vi "03-without_args_and_returned_val.vi"() -> ()   [LabVIEW 2018, in "LV2Julia_examples.lvlib"]
uses:
  LV2Julia_examples.lvlib
  LV2Julia_core/VIs/Server or client state.ctl
  LV2Julia_core/VIs/detailed error info.ctl
  LV2Julia_core/VIs/StackFrame.ctl
  LV2Julia_core/VIs/Commands.ctl
  3a82b6dd-e193-42c5-8b03-f24c274193dd.vi
  3a82b6dd-e193-42c5-8b03-f24c274193dd.vi/3e2a5918-f46e-4ed7-8eb4-9a38b8d3556b.vi
  3a82b6dd-e193-42c5-8b03-f24c274193dd.vi/3e2a5918-f46e-4ed7-8eb4-9a38b8d3556b.vi/37087407-fbe7-4cab-bfef-745450405fa8.vi
  3a82b6dd-e193-42c5-8b03-f24c274193dd.vi/3e2a5918-f46e-4ed7-8eb4-9a38b8d3556b.vi/0226fe71-458f-479f-9501-f13c7d1721aa.vi
  3a82b6dd-e193-42c5-8b03-f24c274193dd.vi/3e2a5918-f46e-4ed7-8eb4-9a38b8d3556b.vi/25bfc6ec-1543-4893-b8db-c428feecb175.vi
  LV2Julia_core/VIs/jl-scripts path.vi
  LV2Julia_core/VIs/check ID validity.vi
  LV2Julia_core/VIs/bindata_descr to JSON.vi
  LV2Julia_core/VIs/check cluster field names.vi
  LV2Julia_core/VIs/concat JSON.vi
  LV2Julia_core/VIs/build request.vi
  LV2Julia_core/VIs/Parse server response.vi
  LV2Julia_core/VIs/log jl exceptions.vi
  LV2Julia_core/LV2Julia_core.lvlib
panel:
  in  "next":bool
  out "detailed error info":T1
  out "current error":errorcluster
  out "final error":errorcluster
  out "short err code":u8
  in  "stop":bool
  out "ZMQ timeout":bool
  out "Julia script file path":path
  out "temporary script path":path
  out "Jl Server state":T3
  # "No arguments are sent and no values recieved here. The Julia script should each time print \"Hello World!\" in the terminal window."
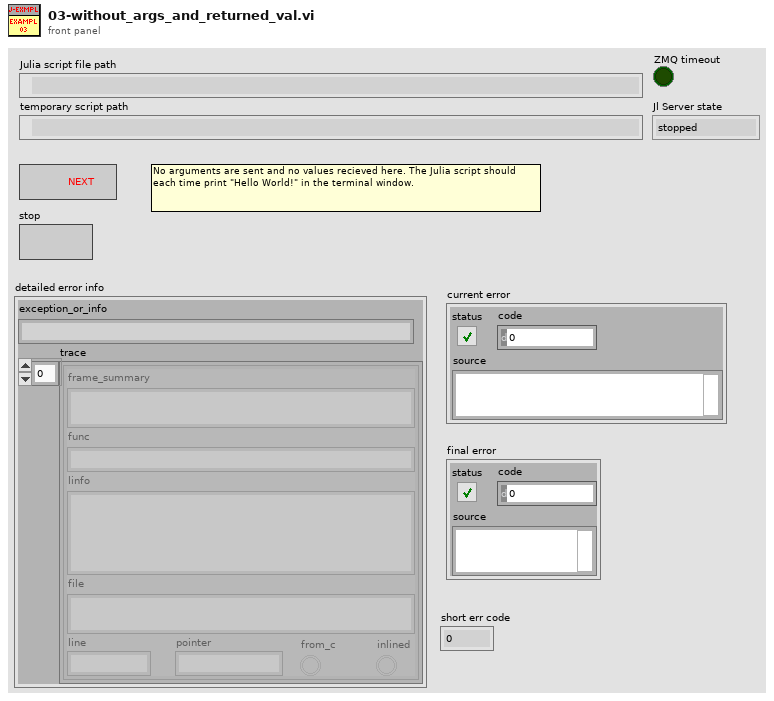
[diagram p1: front panel]
types:
  T1 = typedef "LV2Julia_core.lvlib/detailed error info.ctl" = cluster{"exception_or_info":string, "trace":T2[]}
  T2 = typedef "LV2Julia_core.lvlib/StackFrame.ctl" = cluster{"frame_summary":string, "func":string, "linfo":string, "file":string, "line":i32, "pointer":u64, "from_c":bool, "inlined":bool}
  T3 = typedef "LV2Julia_core.lvlib/Server or client state.ctl" = enum16{"stopped", "running", "unknown"}
  T4 = typedef "LV2Julia_core.lvlib/Commands.ctl" = enum16{"Start Jl-server & Init LV-client", "Send request & Get response ", "Stop Jl-server & Cleanup LV-client", "Cleanup LV-client", "Start Jl-server", "Stop Jl-server", "Init LV-Client", "Cleanup LV-Client", "(not allowed)", "Set LV Client state", "Set Jl Server state", "set ZMQ timeout", "read ZMQ timeout", "read-out state"}
  T5 = typedef "Server state info.ctl" = cluster{"detailed error info":T1, "return code":u8, "Jl Server state":T3}
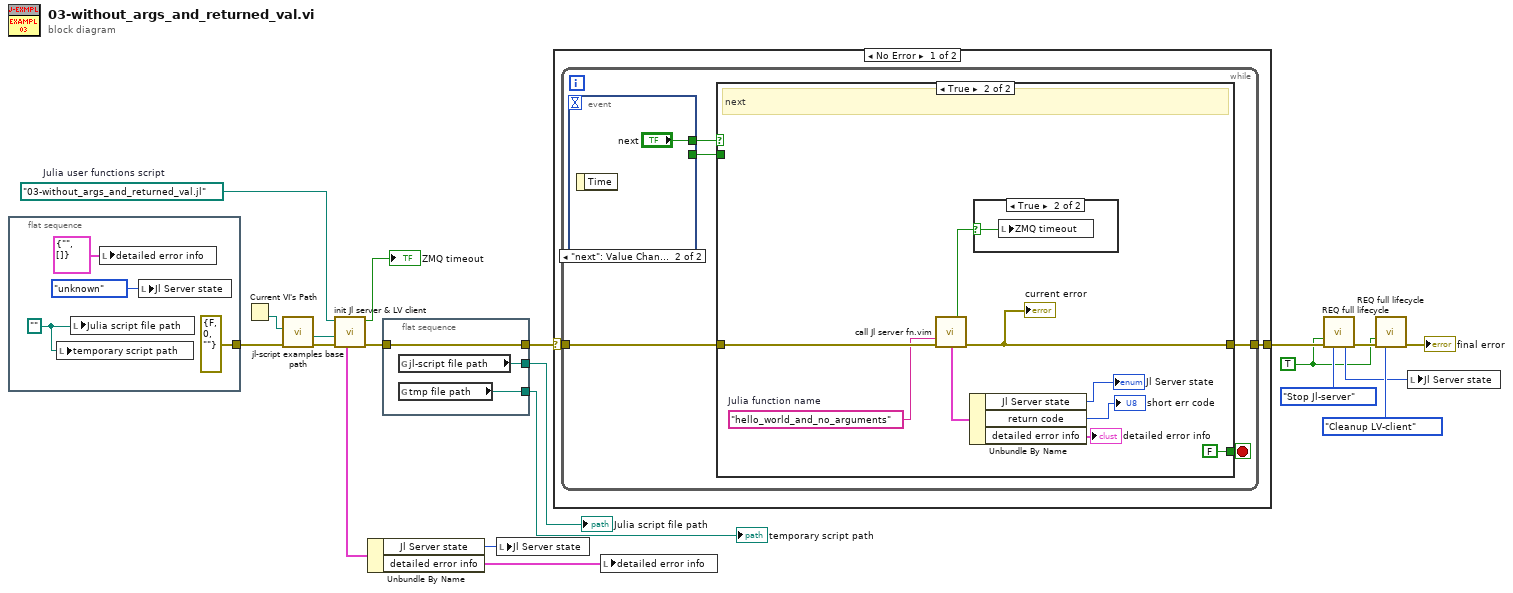
[diagram p0: block diagram]
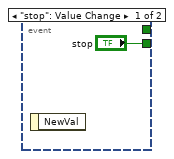
[diagram p2: hidden frame]
diagram:
  w10 = path "03-without_args_and_returned_val.jl"  # Julia user functions script
  w11 = TRUE ("Force command")
  n1 = flat-sequence {
    tunnel: [errorcluster {"status"=FALSE, "code"=0, "source"=""} ("error in (no error)")] -> w4
    frame #0 {
      w21 = path ""
      n2 = local write "temporary script path"(w21) -> ()
      n3 = local write "Julia script file path"(w21) -> ()
      n4 = local write "detailed error info"(T1 {"exception_or_info"="", "trace"=[]} ("detailed error info")) -> ()
      n5 = local write "Jl Server state"(Server_or_client_state."unknown" ("Jl Server state out")) -> ()
    }
  }
  n6 = Current VI's Path() -> (path=w7:path)
  n7 = call "jl-script examples base path.vi"("error in (no error)"=w4, "calling example VI path"=w7) -> ("error out"=w6:errorcluster, "jl-script-examples base path"=w5:path)  [unwired: 8 in]
  n8 = call "init Jl server & LV client.vi"("error in (no error)"=w6, "Base path (not a path)"=w5, "Julia user functions script"=w10) -> ("error out"=w9:errorcluster, "timeout?"=→"ZMQ timeout":bool, "Server state info"=w3:T5)  [unwired: 5 in, 1 out]
  n9 = Unbundle By Name(w3) -> ("Jl Server state"=w1:T3, "detailed error info"=w2:T1)
  n10 = flat-sequence {
    tunnel: [w27] -> w15
    tunnel: w9 -> [w27]
    tunnel: [w26] -> w13
    tunnel: [w25] -> w14
    frame #0 {
      n11 = global read "jl-scripts path.vi" "jl-script file path"() -> (w26:path)
      n12 = global read "jl-scripts path.vi" "tmp file path"() -> (w25:path)
    }
  }
  n13 = local write "Jl Server state"(w1) -> ()
  n14 = case shown="No Error" w15 {
    selector: w15 -> [w28 w49]
    tunnel: [w29 w49] -> w20
    frame No Error {
      n15 = while {
        tunnel: w28 -> [w33]
        tunnel: [w34] -> w29
        stop <- w31 stop-if-true
        n16 = event shown="[1] \"next\": Value Change" {
          selector: _ -> [_ _]
          dyn-events: _ -> [_ _]
          timeout: _ -> [_ _]
          tunnel: [_ "next"] -> w32
          tunnel: ["stop" _] -> w30
          event "stop": Value Change {
            n17 = event-data() -> ()  [unwired: 1 in, 1 out]
          }
          event "next": Value Change {
            n18 = event-data() -> ()  [unwired: 1 in, 1 out]
          }
        }
        n19 = case shown="True" w32 {
          tunnel: [w38 w45] -> w34
          tunnel: w33 -> [w38 w46]
          tunnel: [w37 FALSE ("stop this VI only")] -> w31
          tunnel: w30 -> [w37 _]
          frame False {
            # "stop"
          }
          frame True {
            w43 = "hello_world_and_no_arguments"  # Julia function name
            # "next"
            n20 = call "call Jl server fn.vim"("fun2call"=w43, "error in (no error)"=w46) -> ("timeout?"=w44:bool, "Server state info"=w42:T5, "error out"=w45:errorcluster)  [unwired: 9 in, 2 out]
            "current error" <- w45
            n21 = Unbundle By Name(w42) -> ("Jl Server state"=→"Jl Server state":T3, "return code"=→"short err code":u8, "detailed error info"=→"detailed error info":T1)
            n22 = case shown="True" w44 {
              selector: w44 -> [_ w48]
              frame False {
              }
              frame True {
                n23 = local write "ZMQ timeout"(w48) -> ()
              }
            }
          }
        }
      }
    }
    frame Error {
    }
  }
  n24 = local write "detailed error info"(w2) -> ()
  n25 = call "REQ full lifecycle.vi"("Force command"=w11, "error in"=w20, "command"=Commands."Stop Jl-server") -> ("Jl Server state out"=w12:T3, "error out"=w18:errorcluster)  [unwired: 6 in, 5 out]
  n26 = call "REQ full lifecycle.vi"("Force command"=w11, "error in"=w18, "command"=Commands."Cleanup LV-client") -> ("error out"=→"final error":errorcluster)  [unwired: 6 in, 6 out]
  n27 = local write "Jl Server state"(w12) -> ()
  "temporary script path" <- w14
  "Julia script file path" <- w13
